vi "get AC test parameters.vi"(8 "error in (no error)":errorcluster, 10 "Step":T2=1 min=1 max=99 step=1, 11 "VISA Refnum in":refnum<visa-resource-name>) -> (0 "error out":errorcluster, 3 "VISA Refnum out":refnum<visa-resource-name>, 5 "AC Parameters":T1 {"Voltage Level [V]" min=50 max=5000 step=1 format="%.3p"; "Hi Limit [A]" min=0.0001 max=0.03 step=1e-07 format="%.3p"; "Test Time [s]" min=0.0 max=999.0 step=0.1 format="%.1p"; "Lo Limit [A]" min=0.0 max=0.03 step=1e-07 format="%.3p"; "ARC Limit [A]" min=0.0 max=15.0 format="%.1p"; "Ramp Time [s]" min=0.0 max=999.0 step=0.1 format="%.1p"; "Fall Time [s]" min=0.0 max=999.0 step=0.1 format="%.1p"})   [LabVIEW 2025]
uses:
  <instrlib>/Chrome 19025/Public/Utility/Type Def/steps--numeric.ctl
  AC parameters--cluster.ctl
  <instrlib>/Chrome 19025/Public/Utility/Type Def/AC-DC modes--ring.ctl
  <instrlib>/Chrome 19025/Public/Utility/Type Def/AC-DC-IR modes--ring.ctl
  <instrlib>/Chrome 19025/Chrome 19025.lvlib
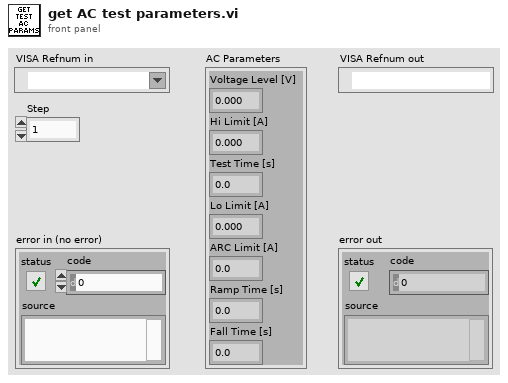
[diagram p1: front panel]
types:
  T1 = typedef "AC parameters--cluster.ctl" = cluster{"Voltage Level [V] ":u16, "Hi Limit [A]":dbl, "Test Time [s] ":dbl, "Lo Limit [A]":dbl, "ARC Limit [A]":dbl, "Ramp Time [s] ":dbl, "Fall Time [s]":dbl}
  T2 = typedef "Chrome 19025.lvlib/steps--numeric.ctl" = u8
  T3 = typedef "Chrome 19025.lvlib/AC-DC modes--ring.ctl" = i32
  T4 = typedef "Chrome 19025.lvlib/AC-DC-IR modes--ring.ctl" = u16
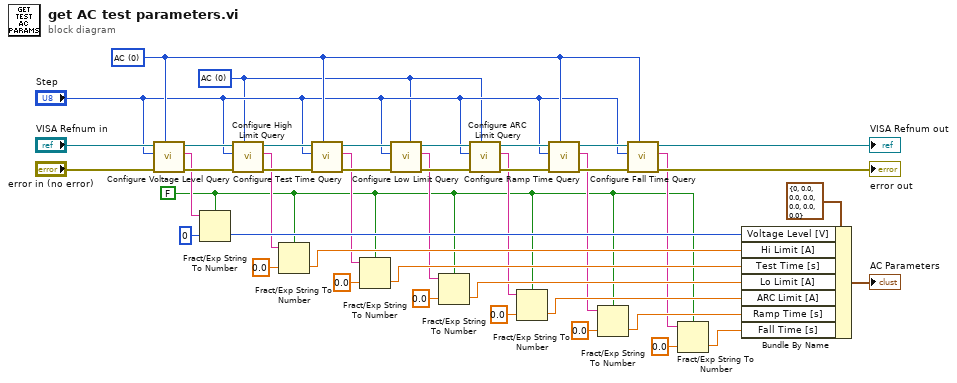
[diagram p0: block diagram]
diagram:
  w2 = FALSE ("use system decimal point (T)")
  w7 = T3 0 items=["AC", "DC"] ("Mode")
  w29 = T4 0 items=["AC", "DC", "IR"] ("Mode")
  n1 = call <instrlib>:"Configure Voltage Level Query.vi"("Mode"=w29, "error in (no error)"="error in (no error)", "Step"="Step", "VISA resource name"="VISA Refnum in") -> ("error out"=w35:errorcluster, "Voltage value [V]"=w25:string, "VISA resource name out"=w32:refnum<visa-resource-name>)  [unwired: 5 in]
  n2 = Fract/Exp String To Number(use system decimal point (T)=w2, string=w25, default (0 dbl)=u16 0 ("Voltage Level [V]")) -> (number=w23:u16)  [unwired: 1 in, 1 out]
  n3 = call <instrlib>:"Configure High Limit Query.vi"("Mode"=w7, "error in (no error)"=w35, "Step"="Step", "VISA resource name"=w32) -> ("error out"=w42:errorcluster, "High value [A]"=w19:string, "VISA resource name out"=w43:refnum<visa-resource-name>)  [unwired: 5 in]
  n4 = Fract/Exp String To Number(use system decimal point (T)=w2, string=w19, default (0 dbl)=0.0) -> (number=w18:dbl)  [unwired: 1 in, 1 out]
  n5 = call <instrlib>:"Configure Test Time Query.vi"("Mode"=w29, "error in (no error)"=w42, "Step"="Step", "VISA resource name"=w43) -> ("error out"=w31:errorcluster, "Test Time value [s]"=w12:string, "VISA resource name out"=w30:refnum<visa-resource-name>)  [unwired: 5 in]
  n6 = Fract/Exp String To Number(use system decimal point (T)=w2, string=w12, default (0 dbl)=0.0) -> (number=w11:dbl)  [unwired: 1 in, 1 out]
  n7 = call <instrlib>:"Configure Low Limit Query.vi"("Mode"=w7, "error in (no error)"=w31, "Step"="Step", "VISA resource name"=w30) -> ("error out"=w36:errorcluster, "Low value [A]"=w6:string, "VISA resource name out"=w37:refnum<visa-resource-name>)  [unwired: 5 in]
  n8 = Fract/Exp String To Number(use system decimal point (T)=w2, string=w6, default (0 dbl)=0.0) -> (number=w10:dbl)  [unwired: 1 in, 1 out]
  n9 = call <instrlib>:"Configure ARC Limit Query.vi"("Mode"=w7, "error in (no error)"=w36, "Step"="Step", "VISA resource name"=w37) -> ("error out"=w38:errorcluster, "ARC Limit value [A]"=w5:string, "VISA resource name out"=w40:refnum<visa-resource-name>)  [unwired: 5 in]
  n10 = Fract/Exp String To Number(use system decimal point (T)=w2, string=w5, default (0 dbl)=0.0) -> (number=w9:dbl)  [unwired: 1 in, 1 out]
  n11 = call <instrlib>:"Configure Ramp Time Query.vi"("Mode"=w29, "error in (no error)"=w38, "Step"="Step", "VISA resource name"=w40) -> ("error out"=w39:errorcluster, "Ramp Time value [s]"=w4:string, "VISA resource name out"=w41:refnum<visa-resource-name>)  [unwired: 5 in]
  n12 = Fract/Exp String To Number(use system decimal point (T)=w2, string=w4, default (0 dbl)=0.0) -> (number=w8:dbl)  [unwired: 1 in, 1 out]
  n13 = call <instrlib>:"Configure Fall Time Query.vi"("Mode"=w29, "error in (no error)"=w39, "Step"="Step", "VISA resource name"=w41) -> ("error out"=→"error out":errorcluster, "Fall Time value"=w3:string, "VISA resource name out"=→"VISA Refnum out":refnum<visa-resource-name>)  [unwired: 5 in]
  n14 = Fract/Exp String To Number(use system decimal point (T)=w2, string=w3, default (0 dbl)=0.0) -> (number=w1:dbl)  [unwired: 1 in, 1 out]
  n15 = Bundle By Name(cluster=T1 {"Voltage Level [V] "=0, "Hi Limit [A]"=0.0, "Test Time [s] "=0.0, "Lo Limit [A]"=0.0, "ARC Limit [A]"=0.0, "Ramp Time [s] "=0.0, "Fall Time [s]"=0.0} ("AC Parameters"), "Voltage Level [V]"=w23, "Hi Limit [A]"=w18, "Test Time [s]"=w11, "Lo Limit [A]"=w10, "ARC Limit [A]"=w9, "Ramp Time [s]"=w8, "Fall Time [s]"=w1) -> (→"AC Parameters":T1)
